vi "Get Code Page.vi"(8 "错误输入（无错误）":errorcluster) -> (0 "错误输出":errorcluster, 3 "CodePage":i32)   [LabVIEW 2012, in "Encoding.lvlib"]
uses:
  Encoding.lvlib
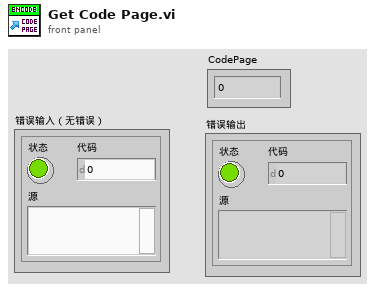
[diagram p1: front panel]
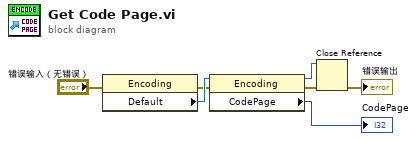
[diagram p0: block diagram]
diagram:
  n1 = property class="Encoding"(error in="错误输入（无错误）") -> (error out=w1:errorcluster, "Default"=w2:refnum<k24>)  [unwired: 1 in, 1 out]
  n2 = property class="Encoding"(reference=w2, error in=w1) -> (reference out=w5:refnum<k24>, error out=w4:errorcluster, "CodePage"=→"CodePage":i32)
  n3 = Close Reference(reference=w5, error in (no error)=w4) -> (error out=→"错误输出":errorcluster)
